vi "误差表格颜色.vi"(8 "合格？":bool, 11 "第几组":i32) -> (2 "颜色":u32)   [LabVIEW 2010]
panel:
  # "0~15"
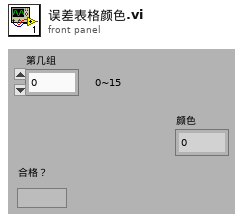
[diagram p1: front panel]
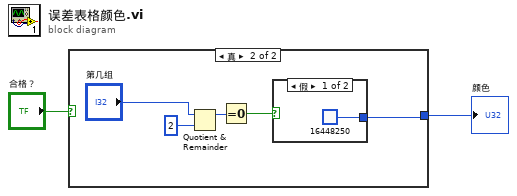
[diagram p0: block diagram]
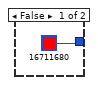
[diagram p2: hidden frame]
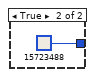
[diagram p3: hidden frame]
diagram:
  n1 = case shown="真" "合格？" {
    tunnel: [u32 16711680 w5] -> w2
    frame False {
    }
    frame True {
      n2 = Quotient & Remainder(x="第几组", y=2) -> (x-y*floor(x/y)=w6:i32)  [unwired: 1 out]
      n3 = Equal To 0?(x=w6) -> (x = 0?=w8:bool)
      n4 = case shown="假" w8 {
        tunnel: [u32 16448250 u32 15723488] -> w5
        frame False {
        }
        frame True {
        }
      }
    }
  }
  "颜色" <- w2
